vi "波形？.vi"() -> ()   [LabVIEW 2017]
panel:
  out "波形图":dbl[](graph)
  in  "波形":enum16{"锯齿", "正弦", "方波", "三角"}(ring)
  in  "振幅":dbl
  in  "频率":dbl
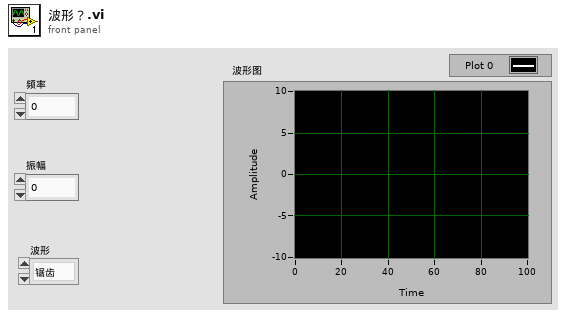
[diagram p1: front panel]
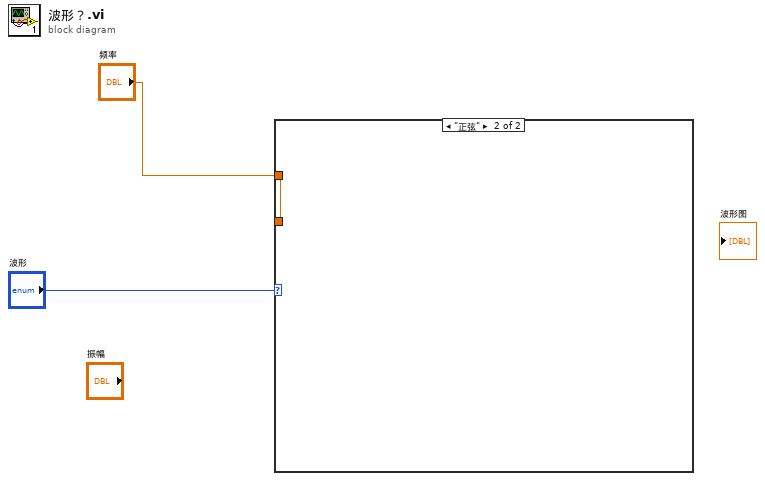
[diagram p0: block diagram]
diagram:
  n1 = case shown="\"正弦\"" "波形" {
    tunnel: [_ w3] -> _
    tunnel: "频率" -> [_ w3]
    frame "锯齿", Default {
    }
    frame "正弦" {
    }
  }
